vi "Obrada podataka.vi"() -> ()   [LabVIEW 2018]
uses:
  <vilib>/Analysis/NI_AALPro.lvlib
panel:
  out "R":dbl
  out "Bez DC":dbl(graph)
  out "Numeric":i32
  out "Trenutni broj otkucaja":i32
  in  "Trajanje merenja pulsa (s)":i32
  out "Izvod":dbl(graph)
  out "Ukupan broj otkucaja":i32
  out "Filtriran":dbl(graph)
  out "Subset 4":dbl[](array[numeric])
  out "Subset 3":dbl[](array[numeric])
  out "Waveform Chart":dbl(graph)
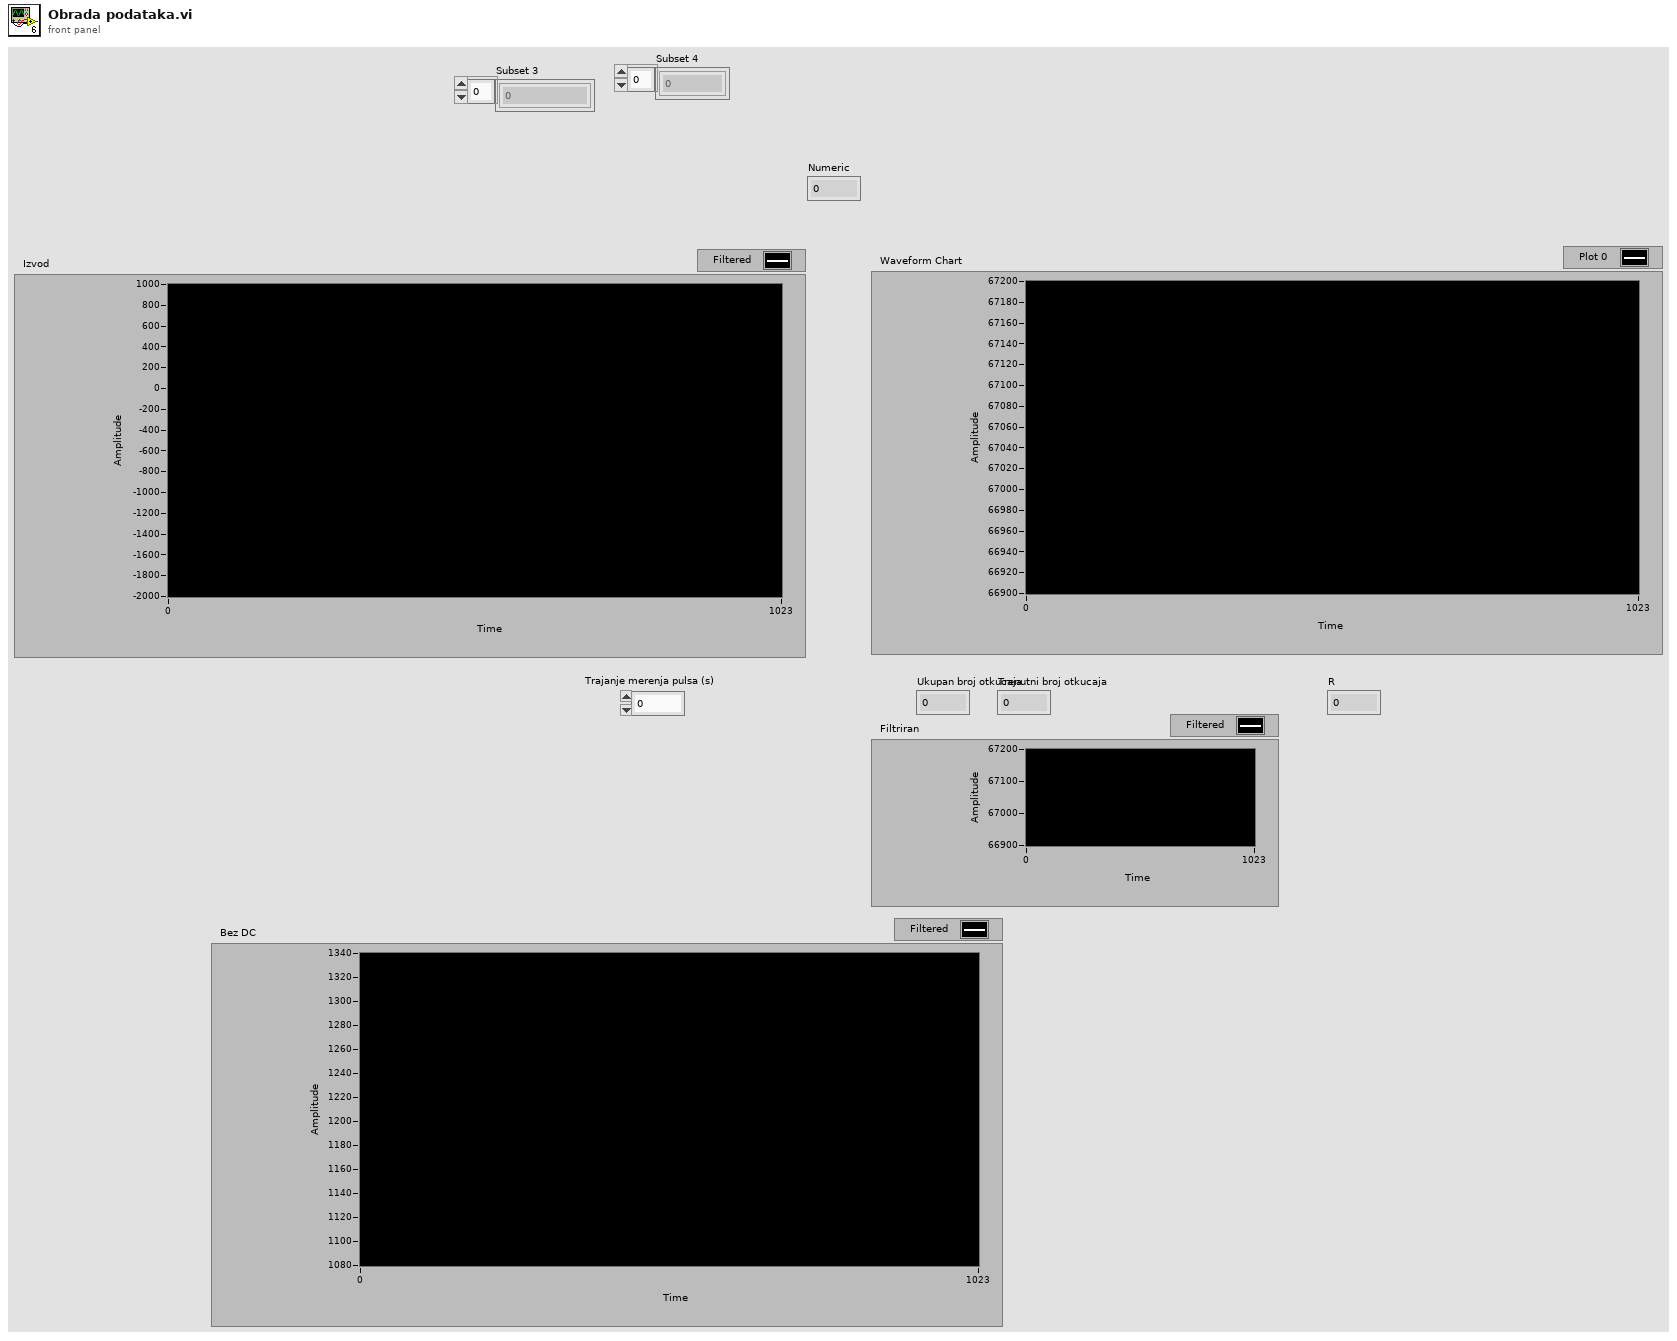
[diagram p1: front panel]
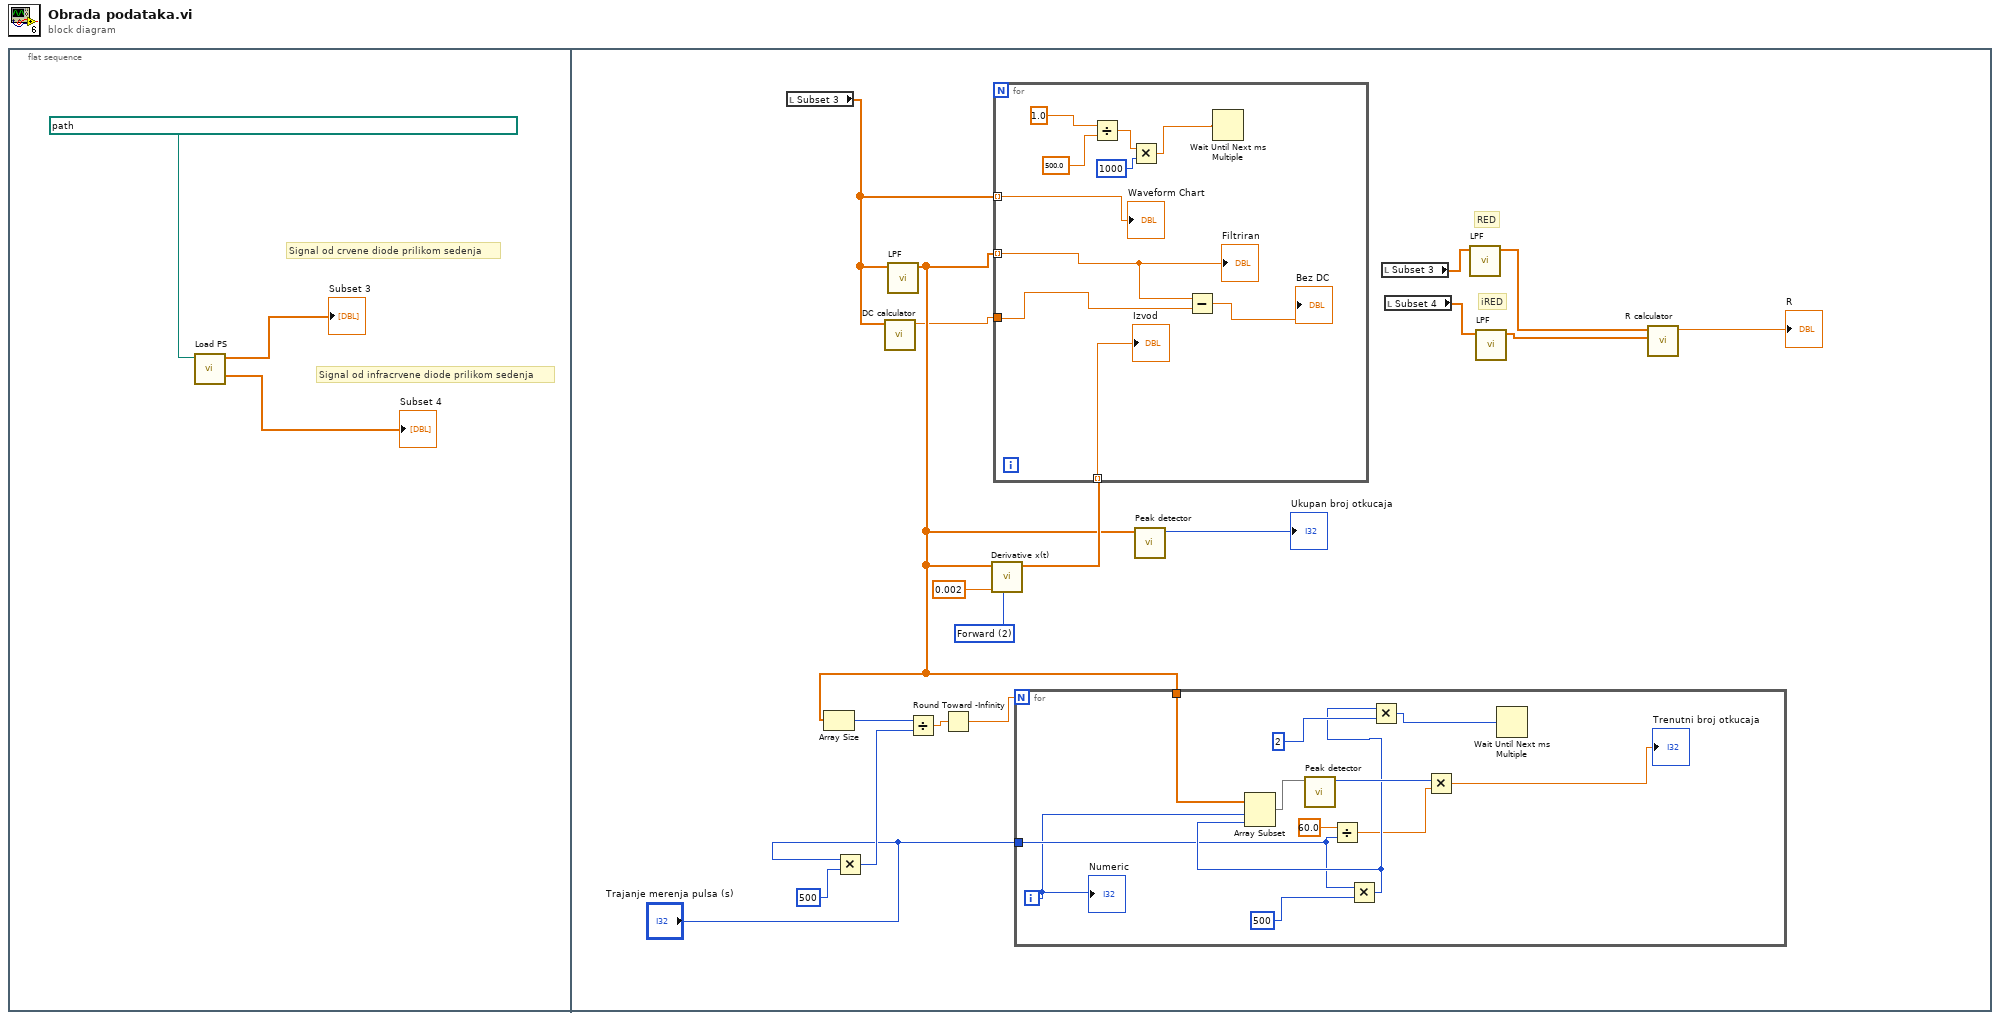
[diagram p0: block diagram]
diagram:
  n1 = flat-sequence {
    frame #0 {
      # "Signal od infracrvene diode prilikom sedenja"
      # "Signal od crvene diode prilikom sedenja"
      n2 = call "Load PS.vi"("Path"=path "C:/Users/djoco/OneDrive/Desktop/Fakultet/4. Godina/8. Semestar/Biomedicinsko inženjerstvo u kognitivnim neuronaukama/Projekat/Data/s10_sit.csv") -> ("Array"=→"Subset 4":dbl[], "Array 2"=→"Subset 3":dbl[])  [unwired: 9 in]
    }
    frame #1 {
      w19 = u16 2 items=["2nd Order Central", "4th Order Central", "Forward", "Backward"] ("method")
      # "iRED"
      # "RED"
      n3 = local read "Subset 3"() -> (w10:dbl[])
      n4 = Multiply(x="Trajanje merenja pulsa (s)", y=500) -> (x*y=w17:i32)
      n5 = call "DC calculator.vi"("Subset 3"=w10) -> ("Numeric"=w9:dbl)  [unwired: 10 in]
      n6 = call "LPF.vi"("Subset 3"=w10) -> ("Filtered X"=w11:dbl[])  [unwired: 10 in]
      n7 = Array Size(array=w11) -> (size(s)=w13:i32)
      n8 = Divide(x=w13, y=w17) -> (x/y=w14:dbl)
      n9 = Round Toward -Infinity(1:w14) -> (0:w15:dbl)
      n10 = call <vilib>:"Derivative x(t).vi"("method"=w19, "dt"=0.002, "X"=w11) -> ("dX/dt"=w18:dbl[])  [unwired: 7 in, 1 out]
      n11 = for {
        tunnel: w10 -> [w43] mode=indexing
        tunnel: w11 -> [w36] mode=indexing
        tunnel: w18 -> [w37] mode=indexing
        tunnel: w9 -> [w35]
        n12 = Divide(x=1.0, y=500.0) -> (x/y=w40:dbl)
        n13 = Multiply(x=w40, y=1000) -> (x*y=w38:dbl)
        n14 = Subtract(x=w36, y=w35) -> (x-y=→"Bez DC":dbl)
        n15 = Wait Until Next ms Multiple(millisecond multiple=w38) -> ()  [unwired: 1 out]
        "Waveform Chart" <- w43
        "Filtriran" <- w36
        "Izvod" <- w37
      }
      n16 = for {
        N: w15 -> [_]
        tunnel: "Trajanje merenja pulsa (s)" -> [w25]
        tunnel: w11 -> [w24]
        i -> [w23]
        n17 = Divide(x=60.0, y=w25) -> (x/y=w26:dbl)
        n18 = Multiply(x=w25, y=500) -> (x*y=w29:i32)
        n19 = Array Subset(array=w24, index=w23, length=w29) -> (w33:dbl[])
        n20 = call "Peak detector.vi"("Filtered X"=w33) -> ("Numeric"=w32:i32)  [unwired: 10 in]
        n21 = Multiply(x=w29, y=2) -> (x*y=w28:i32)
        n22 = Multiply(x=w32, y=w26) -> (x*y=→"Trenutni broj otkucaja":dbl)
        n23 = Wait Until Next ms Multiple(millisecond multiple=w28) -> ()  [unwired: 1 out]
        "Numeric" <- w23
      }
      n24 = call "Peak detector.vi"("Filtered X"=w11) -> ("Numeric"=→"Ukupan broj otkucaja":i32)  [unwired: 10 in]
      n25 = local read "Subset 3"() -> (w7:dbl[])
      n26 = local read "Subset 4"() -> (w8:dbl[])
      n27 = call "LPF.vi"("Subset 3"=w7) -> ("Filtered X"=w6:dbl[])  [unwired: 10 in]
      n28 = call "LPF.vi"("Subset 3"=w8) -> ("Filtered X"=w5:dbl[])  [unwired: 10 in]
      n29 = call "R calculator.vi"("Filtered X"=w5, "Filtered X 2"=w6) -> ("Numeric"=→"R":dbl)  [unwired: 9 in]
    }
  }
